vi "OA Get Number Of Pre Set Modes.vi"(11 "puiNumberOfModes":u32) -> (2 "function return":u32, 3 "puiNumberOfModes out":u32)   [LabVIEW 2018, in "Copy of Andor SDK.lvlib"]
doc: "EXPNETTYPE unsigned int WINAPI OA_GetNumberOfPreSetModes(unsigned int * const puiNumberOfModes);"
uses:
  Copy of Andor SDK.lvlib
  <userlib>/Andor SDK/ATMCD32D.dll
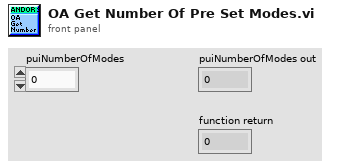
[diagram p1: front panel]
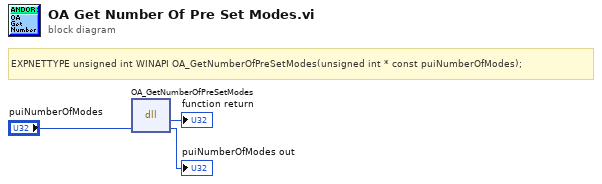
[diagram p0: block diagram]
diagram:
  # "EXPNETTYPE unsigned int WINAPI OA_GetNumberOfPreSetModes(unsigned int * const puiNumberOfModes);"
  n1 = dll-call lib="C:/Program Files (x86)/National Instruments/LabVIEW 2018/user.lib/Andor SDK/ATMCD32D.*" fn="OA_GetNumberOfPreSetModes"("puiNumberOfModes"="puiNumberOfModes") -> (→"function return":u32, "puiNumberOfModes"=→"puiNumberOfModes out":u32)  [unwired: 3 in, 2 out]
